vi "XML Script - Constant.vi"   [LabVIEW 2017]
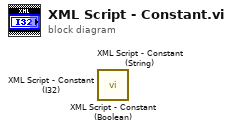
[diagram p0: block diagram]
diagram:
  n1 = call <vilib>:"XML Script - Constant (Boolean).vi"() -> ()  [unwired: 10 in, 2 out]
  n2 = call <vilib>:"XML Script - Constant (String).vi"() -> ()  [unwired: 10 in, 2 out]
  n3 = call <vilib>:"XML Script - Constant (I32).vi"() -> ()  [unwired: 10 in, 2 out]
